vi "Write Testprocess object.vi"(8 "error in (no error)":errorcluster, 10 "Process.lvclass":refnum<class "Process.lvclass">, 11 "Application Test in":refnum<class "Application Test.lvclass">) -> (0 "error out":errorcluster, 3 "Application Test out":refnum<class "Application Test.lvclass">)   [LabVIEW 2020, in "Application Test.lvclass"]
uses:
  Application Test.lvclass
  Framework/Process/Process.lvclass
  Application Test.lvclass/Application Test.ctl
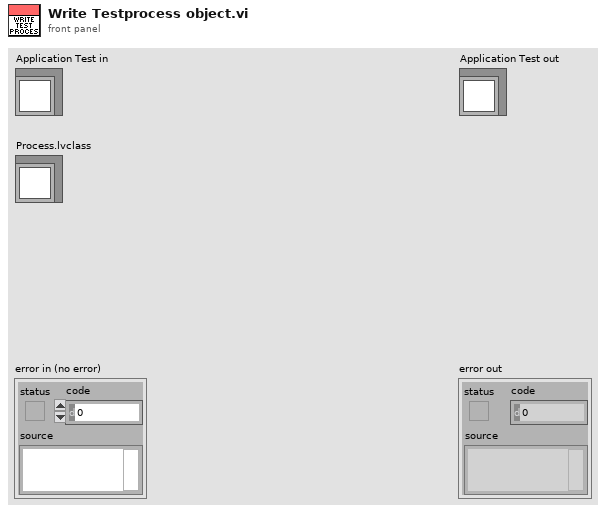
[diagram p1: front panel]
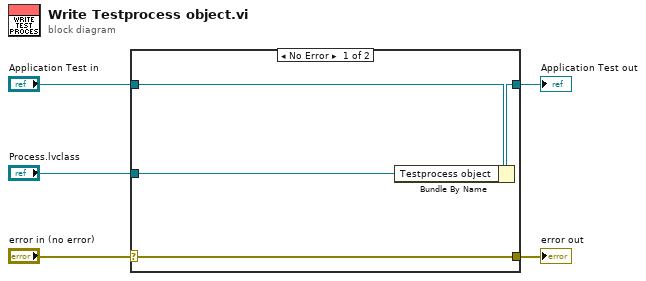
[diagram p0: block diagram]
diagram:
  n1 = case shown="No Error" "error in (no error)" {
    selector: "error in (no error)" -> [w9 w10]
    tunnel: [w9 w10] -> w4
    tunnel: [w7 w11] -> w2
    tunnel: "Application Test in" -> [w8 w11]
    tunnel: "Process.lvclass" -> [w6 _]
    frame No Error {
      n2 = Bundle By Name(cluster=w8, "Testprocess object"=w6) -> (w7:refnum<class "Application Test.lvclass">)
    }
    frame Error {
    }
  }
  "error out" <- w4
  "Application Test out" <- w2
